vi "Write Configuration File.vi"(8 "error in":errorcluster, 11 "Configuration":T1) -> (0 "error out":errorcluster)   [LabVIEW 2020, in "SECS Bridge.lvlib"]
uses:
  SECS Bridge.lvlib
  Configuration.ctl
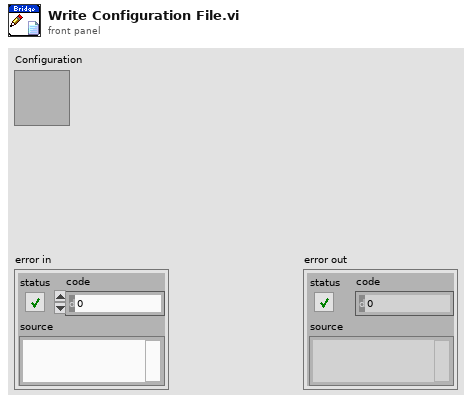
[diagram p1: front panel]
types:
  T1 = typedef "SECS Bridge.lvlib/Configuration.ctl" = cluster{"T3(Reply Timeout)":i32, "T5(Separation Timeout)":i32, "T6(Control Timeout)":i32, "T7(Not Selected Timeout)":i32, "T8(Inter-Character Timeout)":i32, "Session ID":u16, "Log Path":path, "IP Address":string, "Port":u16}
  T2 = enum16{"open", "replace", "create", "open or create", "replace or create", "replace or create with confirmation"}
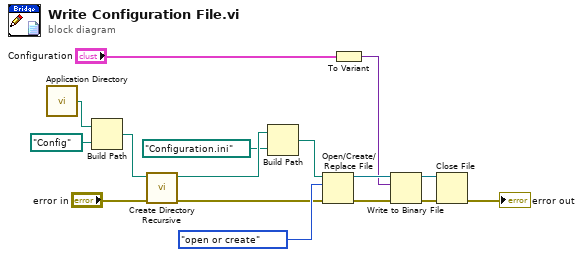
[diagram p0: block diagram]
diagram:
  n1 = call <vilib>:"Application Directory.vi"() -> ("Application Directory"=w16:path)
  n2 = Build Path(base path=w16, name or relative path=path "Config") -> (appended path=w14:path)
  n3 = call <vilib>:"Create Directory Recursive.vi"("error in (no error)"="error in", "directory"=w14) -> ("error out"=w3:errorcluster, "directory copy"=w13:path)  [unwired: 3 in, 1 out]
  n4 = Build Path(base path=w13, name or relative path=path "Configuration.ini") -> (appended path=w2:path)
  n5 = Open/Create/Replace File(file path (use dialog)=w2, error in=w3, operation (0:open)=T2."open or create") -> (refnum out=w9:refnum<file>, error out=w8:errorcluster)  [unwired: 3 in, 1 out]
  n6 = To Variant(anything="Configuration") -> (Variant=w4:variant)
  n7 = Write to Binary File(file (use dialog)=w9, data=w4, error in=w8) -> (refnum out=w7:refnum<file>, error out=w6:errorcluster)  [unwired: 3 in, 1 out]
  n8 = Close File(refnum=w7, error in=w6) -> (error out=→"error out":errorcluster)  [unwired: 1 out]
